vi "NEW File and Save TEST info.vi"(8 "error in":errorcluster caption="Error In", 11 "Test Info":cluster{"Test Name":string, "Tester":string} caption="Test Information Input") -> (0 "error out":errorcluster caption="Error out")   [LabVIEW 2011]
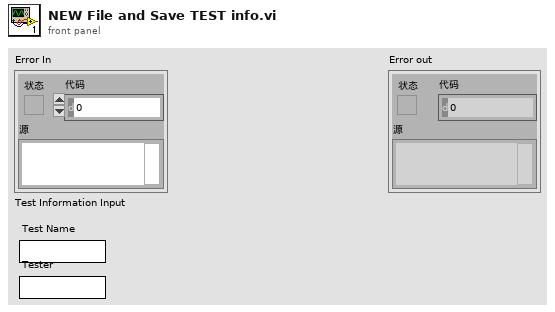
[diagram p1: front panel]
types:
  T1 = typedef "Enum File IO - FGV(V)_Ctrls-某型振动实验台测试系统.ctl" = enum16{"New", "Open", "Write Info", "Write Data", "Read Info", "Read Chan Names", "Read Data", "Close", "None"}
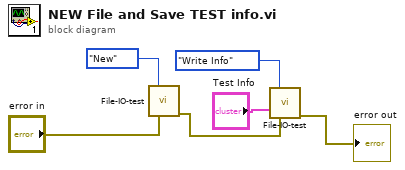
[diagram p0: block diagram]
diagram:
  n1 = call "File-IO-test.vi"("Operation"=Enum_File_IO_-_FGV(V)_Ctrls-某型振动实验台测试系统."New", "error in"="error in") -> ("error out"=w2:errorcluster)  [unwired: 10 in, 3 out]
  n2 = call "File-IO-test.vi"("Operation"=Enum_File_IO_-_FGV(V)_Ctrls-某型振动实验台测试系统."Write Info", "Test Info"="Test Info", "error in"=w2) -> ("error out"=→"error out":errorcluster)  [unwired: 9 in, 3 out]
